vi "ClearHealthAndStatusMemory.vi"(11 "HealthAndStatusSettings":T1={"InternalHealthAndStatusFIFO"="InternalHealthAndStatusFIFO", "HealthAndStatusQueryFIFO"="HealthAndStatusQueryFIFO", "HealthAndStatusResponseFIFO"="HealthAndStatusResponseFIFO", "HealthAndStatusMemory"="HealthAndStatusMemory", "MemorySize"=0}) -> ()   [LabVIEW 2018, in "FPGAHealthAndStatus.lvlib"]
uses:
  FPGAHealthAndStatus.lvlib
  DataTypes/HealthAndStatusSettings.ctl
  <vilib>/rvi/DataTransferAndStorage/Container/Common/niFpgaContainerExecOnDevCompGetState.vi
  <vilib>/rvi/Emulation/niFpgaEmulationIsFPGAContextNoSignature.vi
  <vilib>/rvi/DataTransferAndStorage/Container/Common/niFpgaContainerGetUniqueNameForEmu.vi
  <vilib>/rvi/Emulation/niFpgaProcessEmulError.vi
  <vilib>/rvi/Emulation/niFpgaSctlEmulationGetInTimedLoop.vi
  <vilib>/rvi/errors/nirviReportUnexpectedCaseInternalError (U32).vi
  <vilib>/rvi/Memory/Memory_Emulation/niFpgaMemoryEmulationCacheClearOnFirstRun.vi
  <vilib>/rvi/Memory/Memory_Emulation/nirvimemoryEmulationManagerCache_MakeExclusive.vi
  <vilib>/rvi/Memory/Memory_Emulation/niFpgaMemoryEmulationValidateCache.vi
  <vilib>/rvi/Memory/Memory_Emulation/nirvimemoryEmulationManagerCache_InsertValue.vi
  <vilib>/Utility/error.llb/Clear Errors.vi
  <vilib>/rvi/Memory/Memory_Emulation/nirvimemoryEmulationManagerCache_ReleaseExclusive.vi
  <vilib>/rvi/Memory/Memory_Emulation/nirvimemoryEmulationManagerCache_GetValue.vi
  <vilib>/rvi/Memory/Memory_Emulation/nirvimemoryEmulationManagerCache_SetValue.vi
  <vilib>/rvi/Emulation/niFpgaSctlEmulationResourceMgr.vi
  <vilib>/rvi/DataTransferAndStorage/Container/XNode/niFpgaContainer.xnode
  <vilib>/rvi/Memory/Memory_Emulation/niFpgaMemoryEmulationRefIn.vi
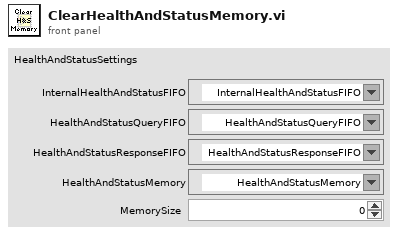
[diagram p1: front panel]
types:
  T1 = typedef "FPGAHealthAndStatus.lvlib/HealthAndStatusSettings.ctl" = cluster{"InternalHealthAndStatusFIFO":refnum<k21>, "HealthAndStatusQueryFIFO":refnum<k21>, "HealthAndStatusResponseFIFO":refnum<k21>, "HealthAndStatusMemory":refnum<k21>, "MemorySize":i32}
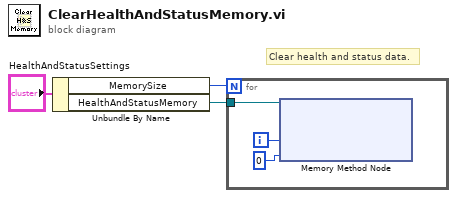
[diagram p0: block diagram]
diagram:
  # "Clear health and status data."
  n1 = Unbundle By Name("HealthAndStatusSettings") -> ("MemorySize"=w2:i32, "HealthAndStatusMemory"=w1:refnum<k21>)
  n2 = for {
    N: w2 -> [_]
    tunnel: w1 -> [w4]
    i -> [w6]
    n3 = xnode ("Memory Method Node")("Address"=w6, "Data"=u64 0, "Memory In"=w4) -> ()  [unwired: 1 out]
  }
